vi "Search 1D String Array.vi"(8 "error in (no error)":errorcluster, 9 "Search String":string, 11 "1D String Array":string[](array[string])) -> (0 "error out":errorcluster, 1 "Found?":bool, 3 "Index":i32)   [LabVIEW 2020, in "FTDI Finder.lvlib"]
uses:
  FTDI Finder.lvlib
  <vilib>/regexp/Match Regular Expression.xnode
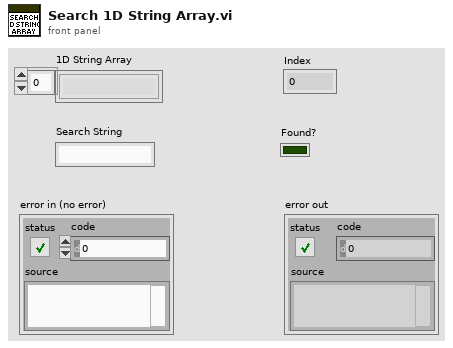
[diagram p1: front panel]
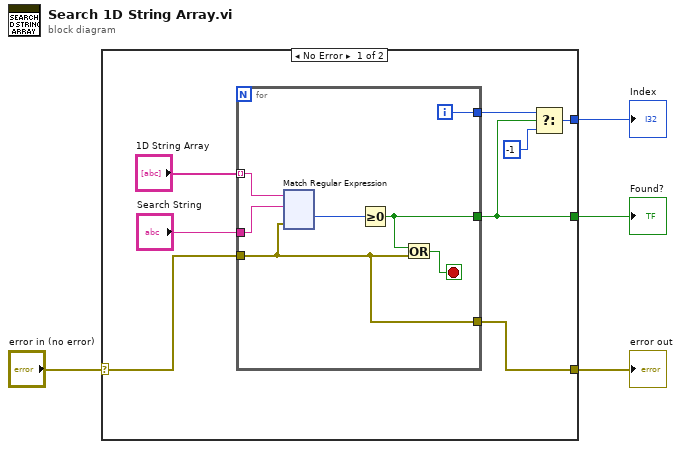
[diagram p0: block diagram]
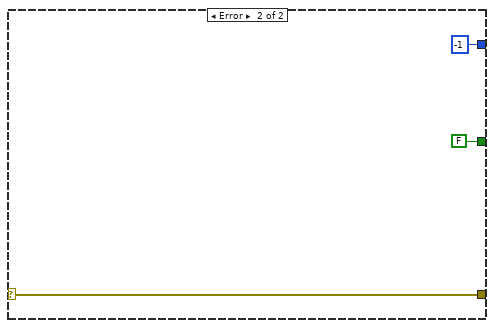
[diagram p2: hidden frame]
diagram:
  n1 = case shown="No Error" "error in (no error)" {
    selector: "error in (no error)" -> [w10 w136]
    tunnel: [w9 w136] -> w3
    tunnel: [w8 FALSE] -> w2
    tunnel: [w5 -1 ("f")] -> w1
    frame No Error {
      n2 = for {
        tunnel: "1D String Array" -> [w19] mode=indexing
        tunnel: "Search String" -> [w18]
        tunnel: w10 -> [w15]
        tunnel: [w15] -> w9
        tunnel: [w14] -> w8
        tunnel: [w13] -> w7
        i -> [w13]
        stop <- w16 stop-if-true
        n3 = xnode "Match Regular Expression"("input string"=w19, "regular expression"=w18, "error in"=w15) -> ("offset past match"=w17:i32)  [unwired: 3 in, 4 out]
        n4 = Greater Or Equal To 0?(x=w17) -> (x >= 0?=w14:bool)
        n5 = Or(x=w14, y=w15) -> (x .or. y?=w16:bool)
      }
      n6 = Select(t=w7, s=w8, f=-1) -> (s? t:f=w5:i32)
    }
    frame Error {
    }
  }
  "Index" <- w1
  "Found?" <- w2
  "error out" <- w3
